vi "IV_Reader_SweepScroller.vi"() -> ()   [LabVIEW 2016]
panel:
  in  "Sweep parameters":T1
  in  "PNG output folder":path=path "C:/Users/ansom/Desktop/Agilent/PNG's From Graphs/B_BG_7to-7"
  in  "Large Sweep Folder":path=path "P:/sample/GaAs/GaAs quantum dots/2008/PL Map/A1 735/060731ASBA_A1_6.0.itx"
  in  "# Fast Sweep":dbl
  in  "# Slow Sweep":dbl
  # "Vbg will be updated autmatically"
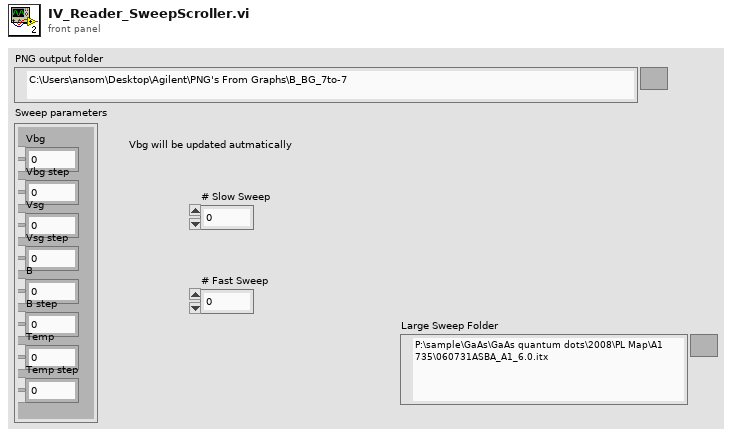
[diagram p1: front panel]
types:
  T1 = cluster{"Vbg":dbl, "Vbg step":dbl, "Vsg":dbl, "Vsg step":dbl, "B":dbl, "B step":dbl, "Temp":dbl, "Temp step":dbl}
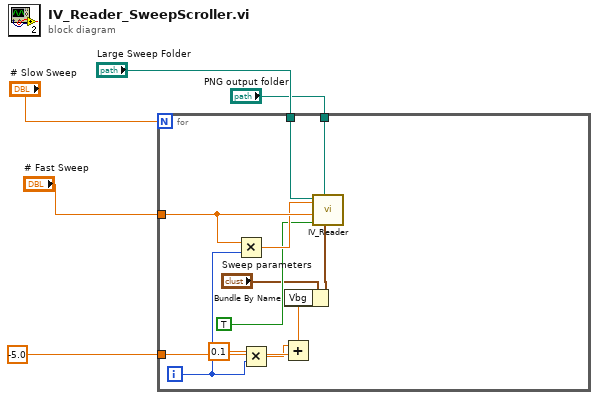
[diagram p0: block diagram]
diagram:
  n1 = for {
    N: "# Slow Sweep" -> [_]
    tunnel: "# Fast Sweep" -> [w17]
    tunnel: "Large Sweep Folder" -> [w15]
    tunnel: "PNG output folder" -> [w13]
    tunnel: -5.0 -> [w8]
    i -> [w9]
    n2 = Multiply(x=w17, y=w9) -> (x*y=w16:dbl)
    n3 = Multiply(x=0.1, y=w9) -> (x*y=w7:dbl)
    n4 = Add(x=w7, y=w8) -> (x+y=w6:dbl)
    n5 = Bundle By Name(cluster="Sweep parameters", "Vbg"=w6) -> (w11:T1)
    n6 = call "IV_Reader.vi"("Sweep parameters"=w11, "Path to PNG Folder"=w13, "Use only a subset of the folder"=TRUE ("Use File Offset"), "Subset Length"=w17, "Subset Index"=w16, "Folder or File"=w15) -> ()  [unwired: 6 in]
  }
